vi "sql test.vi"() -> ()   [LabVIEW 2017]
uses:
  <vilib>/addons/database/Connection.llb/DB Tools Open Connec (Path).vi
  <vilib>/addons/database/_DB Variant To Data/Database Variant To Data.xnode
  <vilib>/addons/database/NI_Database_API.lvlib
panel:
  out "columns 2":string[](array[string])
  out "columns":string[](array[string])
  out "data 3":string[][](array[string])
  in  "error out 2":errorcluster
  out "resulting string":string
  out "data 2":string[][](array[string])
  out "error out":errorcluster
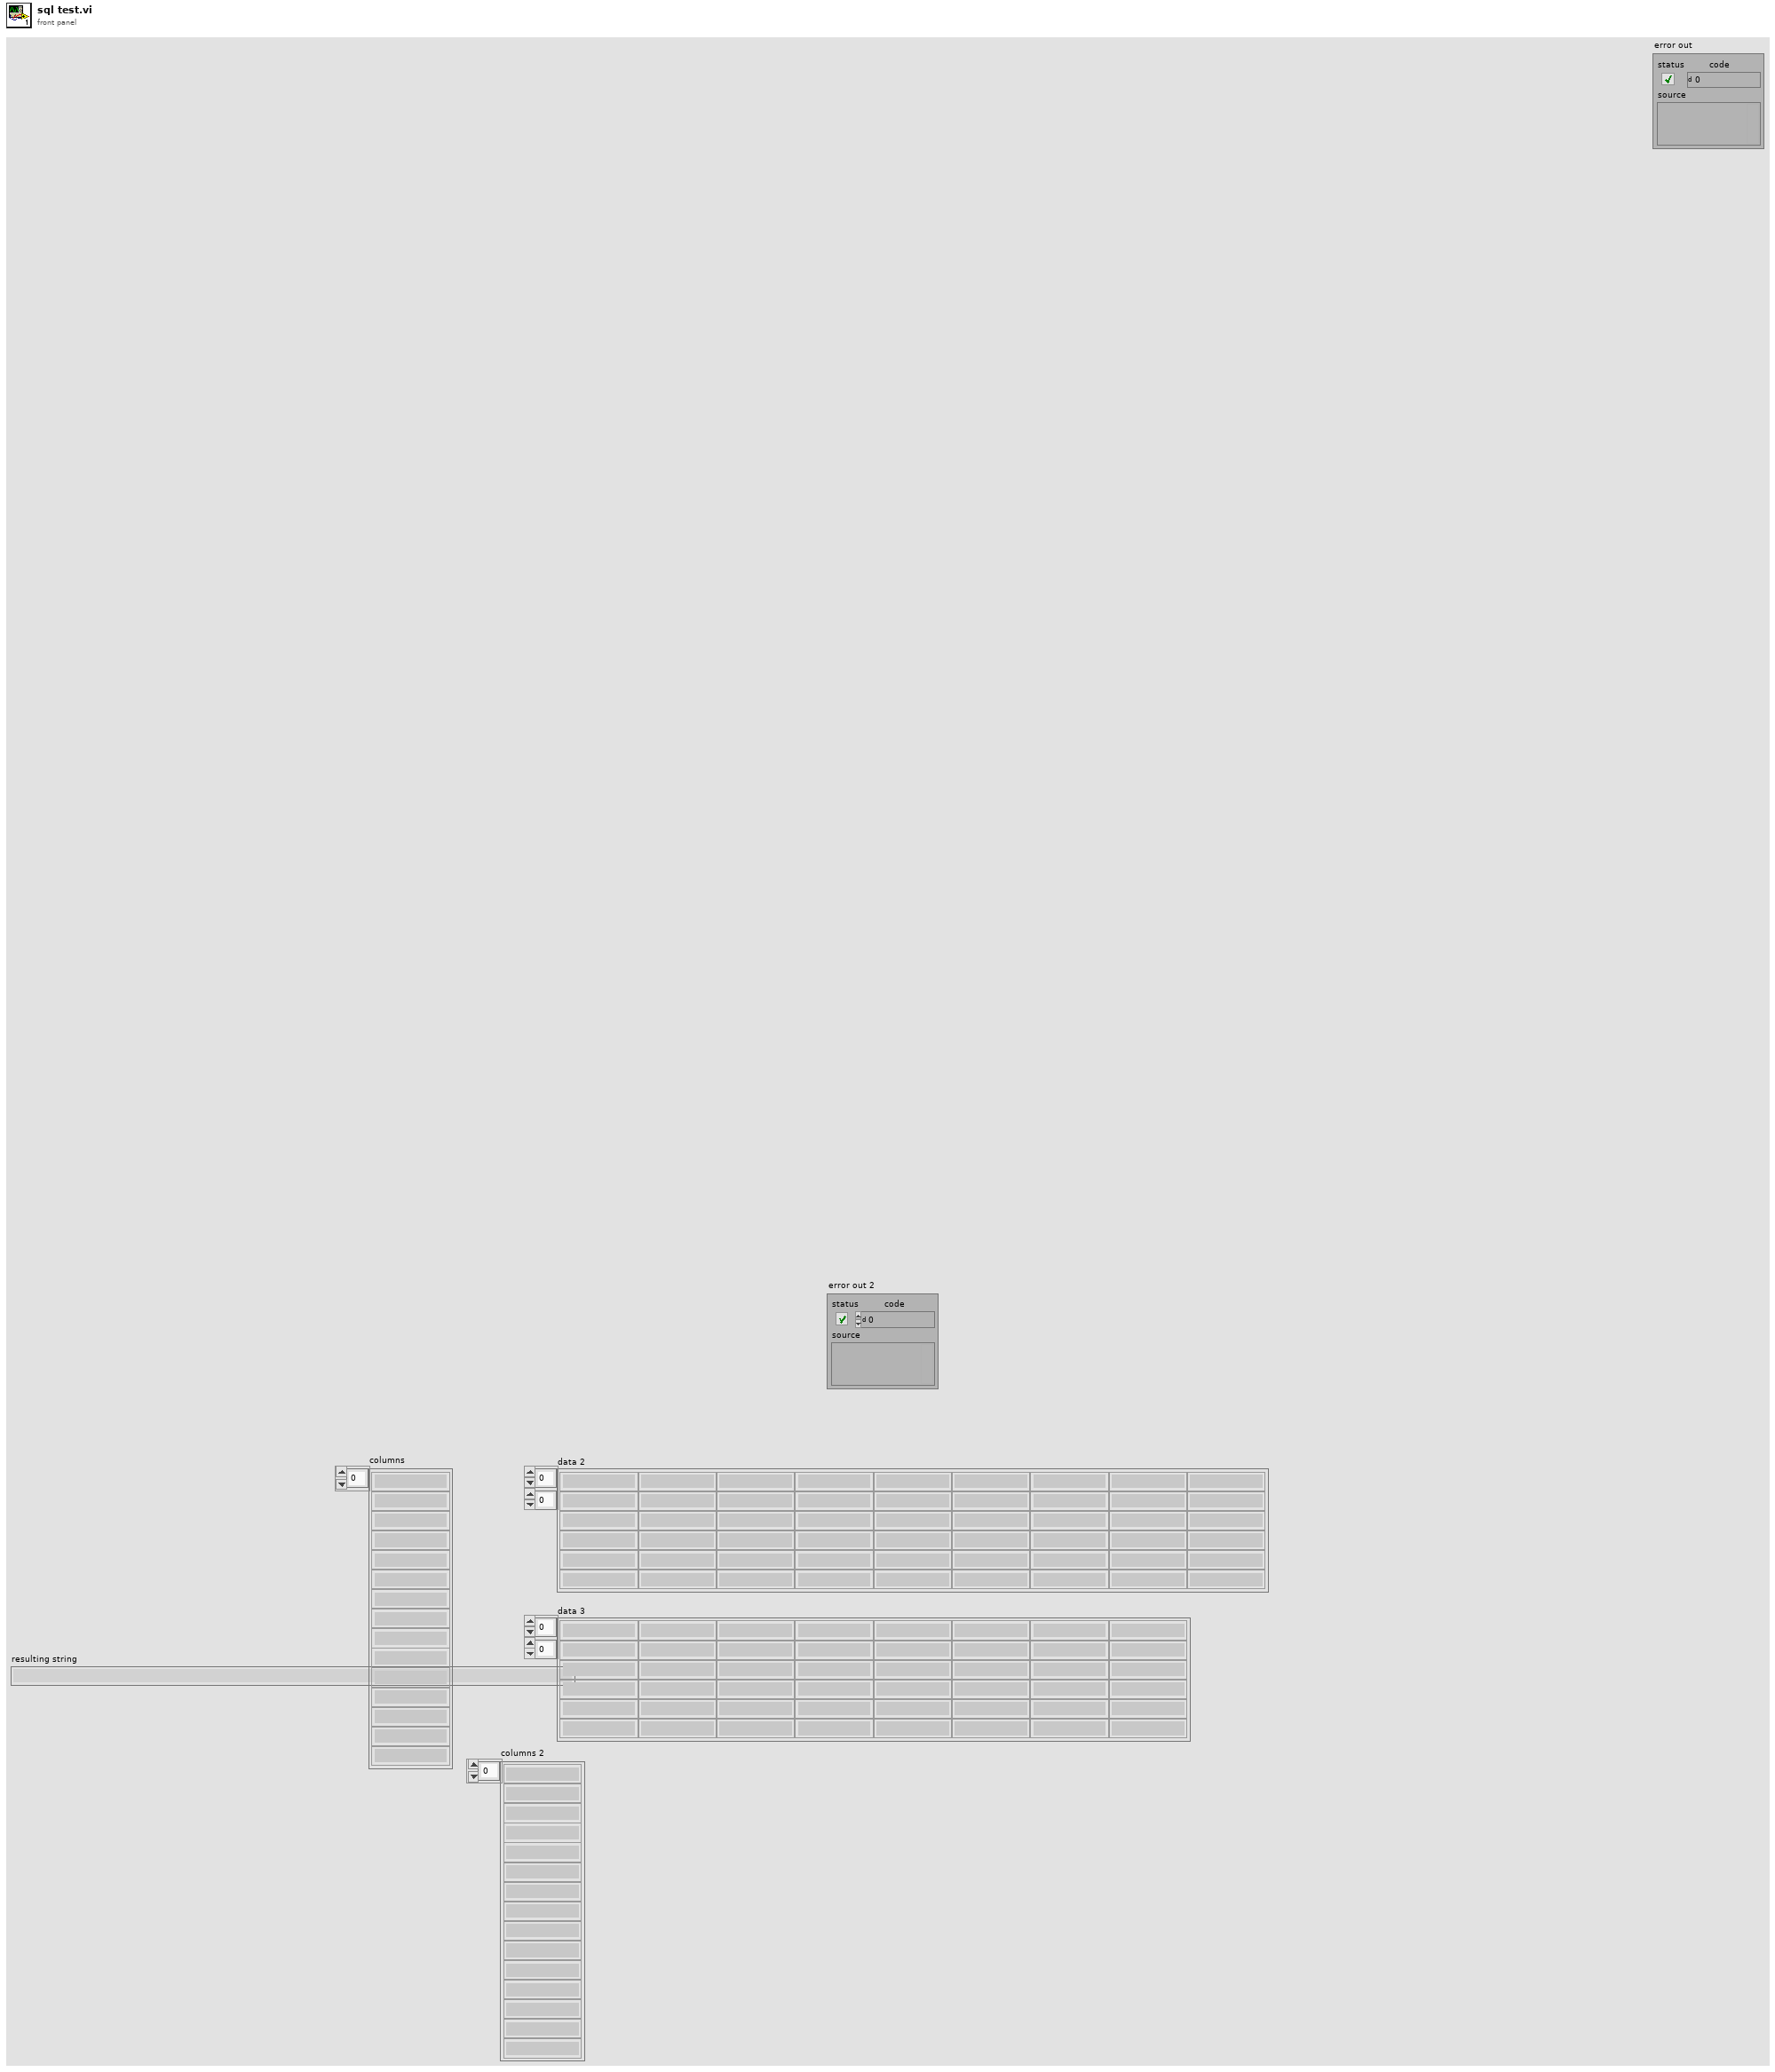
[diagram p1: front panel]
types:
  T1 = typedef "NI_Database_API.lvlib/Conn ObjectReference.ctl" = refnum<k1>
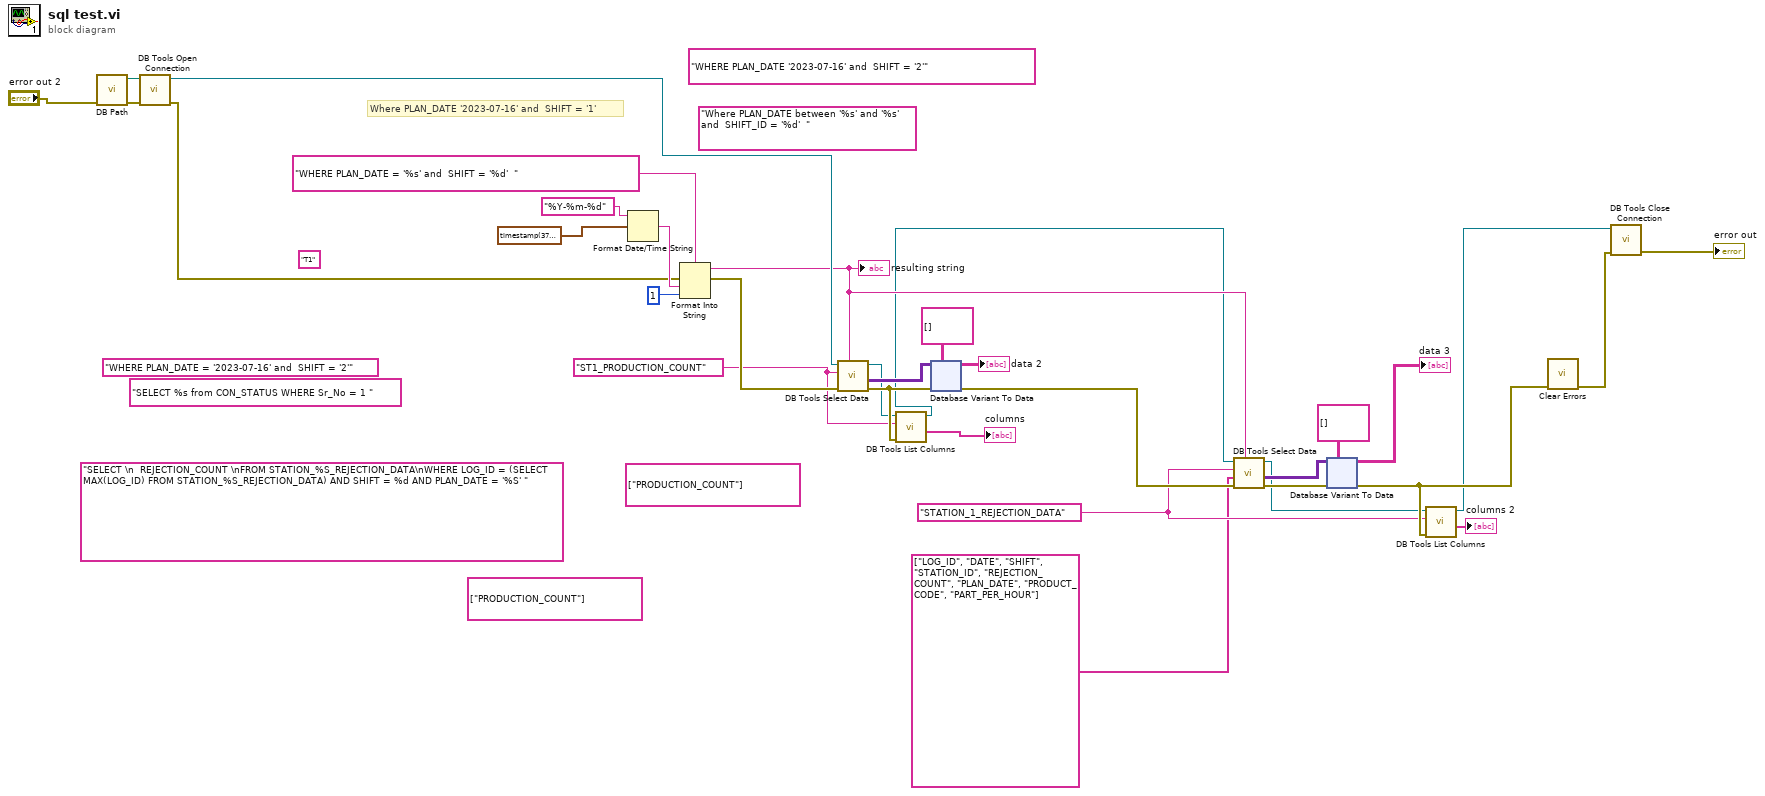
[diagram p0: block diagram]
diagram:
  (unwired) string[] ["PRODUCTION_COUNT"] ("columns")
  w7 = "STATION_1_REJECTION_DATA" ("table")
  (unwired) "SELECT \n  REJECTION_COUNT \nFROM STATION_%S_REJECTION_DATA\nWHERE LOG_ID = (SELECT MAX(LOG_ID) FROM STATION_%S_REJECTION_DATA) AND SHIFT = %d AND PLAN_DATE = '%S' " ("SQL query")
  (unwired) "WHERE PLAN_DATE = '2023-07-16' and  SHIFT = '2'" ("resulting string 2")
  (unwired) "Where PLAN_DATE between '%s' and '%s' and  SHIFT_ID = '%d'  "
  (unwired) "WHERE PLAN_DATE '2023-07-16' and  SHIFT = '2'"
  (unwired) string[] ["PRODUCTION_COUNT"] ("columns")
  w10 = "ST1_PRODUCTION_COUNT" ("table")
  (unwired) "T1"
  (unwired) "SELECT %s from CON_STATUS WHERE Sr_No = 1 " ("SQL query")
  # "Where PLAN_DATE '2023-07-16' and  SHIFT = '1'"
  n1 = call "DB Path.vi"("error in"="error out 2") -> ("error out"=w32:errorcluster, "DB Path"=w33:path)  [unwired: 9 in]
  n2 = call-poly <vilib>:"DB Tools Open Connection.vi"("error in (no error)"=w32, "connection information"=w33) -> ("error out"=w24:errorcluster, "connection reference"=w20:T1)  [unwired: 6 in]
  n3 = Format Date/Time String(time format string (%c)="%Y-%m-%d", seconds (now)=timestamp(3772396800 s since 1904-01-01) ("Date")) -> (date/time string=w27:string)  [unwired: 1 in]
  n4 = Format Into String(format string="WHERE PLAN_DATE = '%s' and  SHIFT = '%d'  ", error in=w24, w27, 1 ("input 2")) -> (resulting string=w13:string, error out=w29:errorcluster)  [unwired: 1 in]
  "resulting string" <- w13
  n5 = call <vilib>:"DB Tools Select Data.vi"("condition"=w13, "error in (no error)"=w29, "table"=w10, "connection reference"=w20) -> ("error out"=w11:errorcluster, "data"=w28:variant[][], "connection reference out"=w6:T1)  [unwired: 2 in]
  n6 = call <vilib>:"DB Tools List Columns.vi"("error in (no error)"=w11, "table"=w10, "connection reference"=w6) -> ("columns"=→"columns":string[], "connection reference out"=w5:T1)  [unwired: 1 in, 2 out]
  n7 = xnode "Database Variant To Data"("database variant"=w28, "error in (no error)"=w11, "type"=string[][] [] ("Elements Found")) -> ("data"=→"data 2":string[][], "error out"=w12:errorcluster)
  n8 = call <vilib>:"DB Tools Select Data.vi"("condition"=w13, "error in (no error)"=w12, "columns"=string[] ["LOG_ID", "DATE", "SHIFT", "STATION_ID", "REJECTION_COUNT", "PLAN_DATE", "PRODUCT_CODE", "PART_PER_HOUR"] ("columns 3"), "table"=w7, "connection reference"=w5) -> ("error out"=w15:errorcluster, "data"=w16:variant[][], "connection reference out"=w4:T1)  [unwired: 1 in]
  n9 = xnode "Database Variant To Data"("database variant"=w16, "error in (no error)"=w15, "type"=string[][] [] ("Elements Found")) -> ("data"=→"data 3":string[][], "error out"=w8:errorcluster)
  n10 = call <vilib>:"DB Tools List Columns.vi"("error in (no error)"=w8, "table"=w7, "connection reference"=w4) -> ("columns"=→"columns 2":string[], "connection reference out"=w3:T1)  [unwired: 1 in, 2 out]
  n11 = call <vilib>:"Clear Errors.vi"("error in (no error)"=w8) -> ("error out"=w19:errorcluster)  [unwired: 5 in, 1 out]
  n12 = call <vilib>:"DB Tools Close Connection.vi"("error in (no error)"=w19, "connection reference"=w3) -> ("error out"=→"error out":errorcluster)  [unwired: 5 in]
